vi "Do Charact.vi"(0 "Scalar Path in":refnum<class "Scalar Path.lvclass">, 5 "Standard Type":T1, 11 "error in (no error)":errorcluster) -> (4 "Scalar Path out":refnum<class "Scalar Path.lvclass">, 6 "Aborted":bool, 15 "error out":errorcluster)   [LabVIEW 2023, in "RFFixtureCharact.Public.lvlib" / "Scalar Path.lvclass"]
uses:
  Scalar Path.lvclass
  C:/srd-semi-rfcal-software/AuxTools/STSRFFixtureCharactUtility/Source/Code Modules/Common/Base Classes/Path/Path.lvclass
  Type Definitions/Cal Point.ctl
  Scalar Path.lvclass/Scalar Path.ctl
  Instruments/Cal Standard/Type Definitions/Standard Type.ctl
  Instruments/RFFixtureCharact.Instruments.lvlib
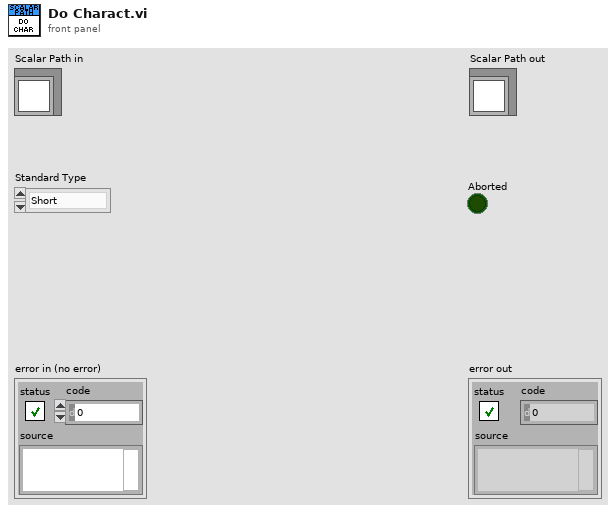
[diagram p1: front panel]
types:
  T1 = typedef "RFFixtureCharact.Instruments.lvlib/Standard Type.ctl" = enum16{"Short", "Open", "Load", "PowerMeter", "None"}
  T2 = typedef "RFFixtureCharact.Public.lvlib/Scalar Path.lvclass/Cal Point.ctl" = cluster{"Port Power":dbl, "Frequency":dbl, "Reference Level":dbl}
  T3 = typedef "RFFixtureCharact.Public.lvlib/Scalar Path Group.lvclass/Sweep.ctl" = cluster{"Port Power":dbl, "Frequencies":dbl[], "Reference Level":dbl}
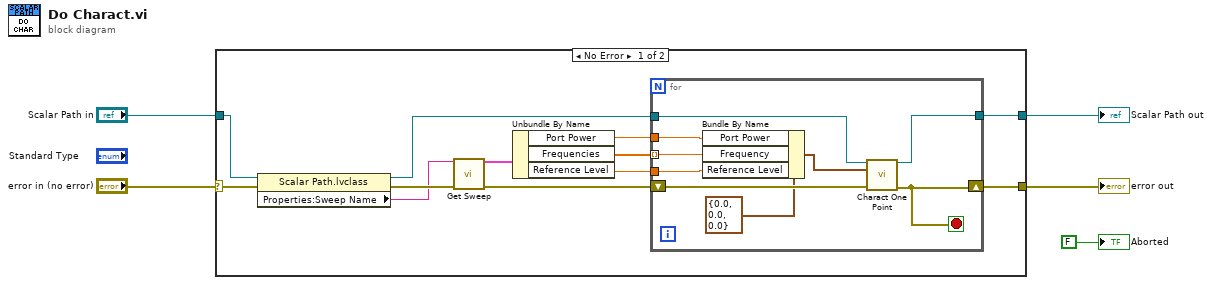
[diagram p0: block diagram]
diagram:
  n1 = case shown="No Error" "error in (no error)" {
    selector: "error in (no error)" -> [w10 w28]
    tunnel: [w11 w28] -> w2
    tunnel: [w12 w27] -> w4
    tunnel: "Scalar Path in" -> [w14 w27]
    frame No Error {
      n2 = property class="Scalar Path.lvclass"(reference=w14, error in=w10) -> (reference out=w13:refnum<class "Scalar Path.lvclass">, error out=w9:errorcluster, "Properties:Sweep Name"=w7:string)
      n3 = call "Get Sweep.vi"("Sweep Name"=w7, "error in (no error)"=w9) -> ("Sweep"=w6:T3, "error out"=w8:errorcluster)  [unwired: 11 in, 1 out]
      n4 = Unbundle By Name(w6) -> ("Port Power"=w17:dbl, "Frequencies"=w15:dbl[], "Reference Level"=w16:dbl)
      n5 = for {
        tunnel: w17 -> [w26]
        tunnel: w16 -> [w25]
        tunnel: w15 -> [w24] mode=indexing
        tunnel: w13 -> [w23]
        tunnel: [w20] -> w12
        shift-right: [w19] -> w11
        shift-left: w8 -> [w22]
        stop <- w19 stop-if-true
        n6 = Bundle By Name(cluster=T2 {"Port Power"=0.0, "Frequency"=0.0, "Reference Level"=0.0} ("Cal Point"), "Port Power"=w26, "Frequency"=w24, "Reference Level"=w25) -> (w21:T2)
        n7 = call-dynamic "Charact One Point.vi"("Scalar Path in"=w23, "Cal Point in"=w21, "error in (no error)"=w22) -> ("Scalar Path out"=w20:refnum<class "Scalar Path.lvclass">, "error out"=w19:errorcluster)  [unwired: 11 in]
      }
    }
    frame Error {
    }
  }
  "error out" <- w2
  "Scalar Path out" <- w4
  "Aborted" <- FALSE ("If Aborted")
